vi "Stage position constant read.vi"(11 "Queue in":refnum<queue>) -> ()   [LabVIEW 2020]
panel:
  out "Stage position":dbl format="%.1f"
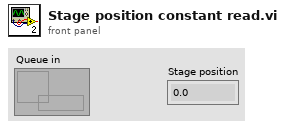
[diagram p1: front panel]
types:
  T1 = enum32{"invalid app kind", "Development System", "Run Time System", "Student Edition", "Embedded LabVIEW", "Evaluation", "Custom"}
  T2 = enum32{"Invalid", "Standard", "Closed", "Hidden", "Minimized", "Maximized"}
  T3 = cluster{"Core":cluster{"Current VI Reference":refnum<vi>, "Close Panel on Exit?":bool}, "Stage name":string, "Stage variable name":string, "Stage TCP":refnum<k5>, "Stage status":cluster{"stage position":dbl, "display error":bool}, "connected":bool}
  T4 = cluster{"stage position":dbl, "display error":bool}
  T5 = cluster{"Current VI Reference":refnum<vi>, "Close Panel on Exit?":bool}
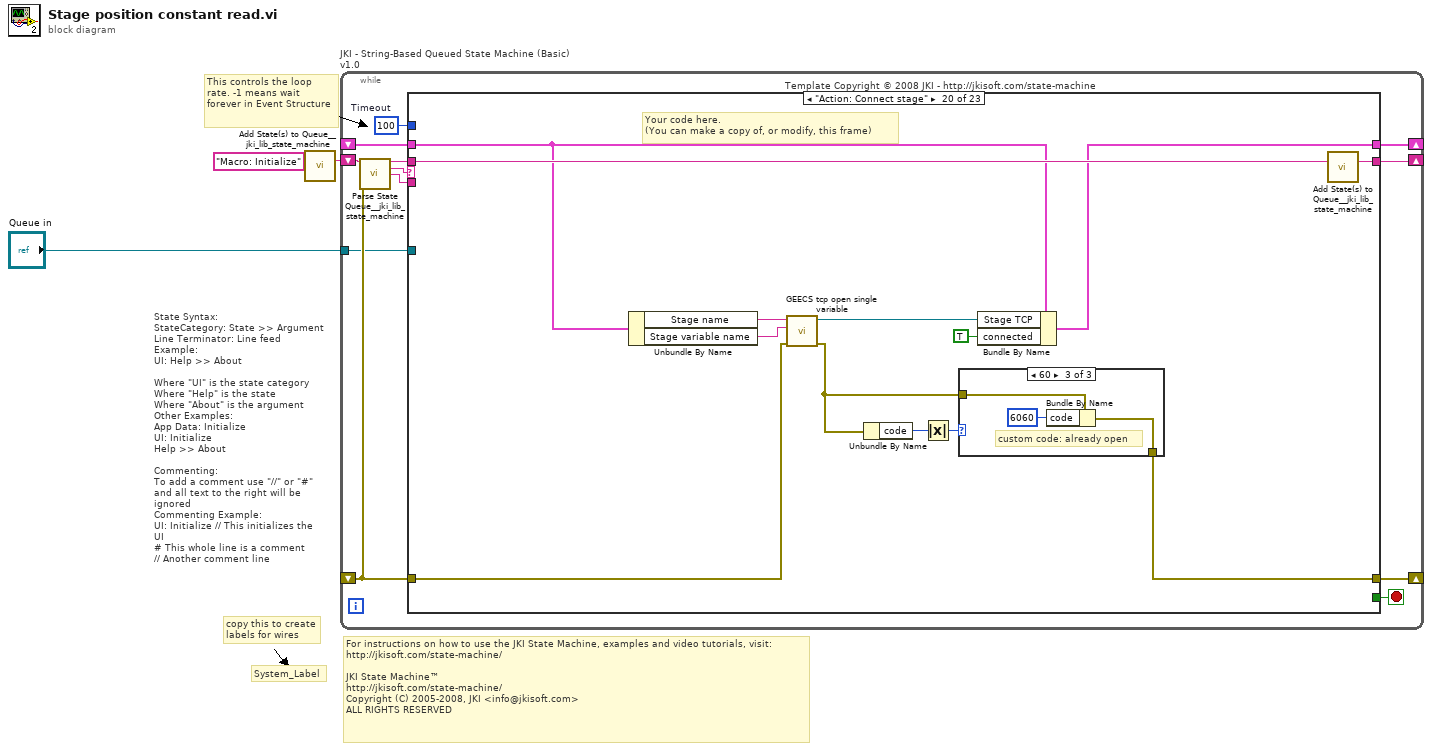
[diagram p0: block diagram]
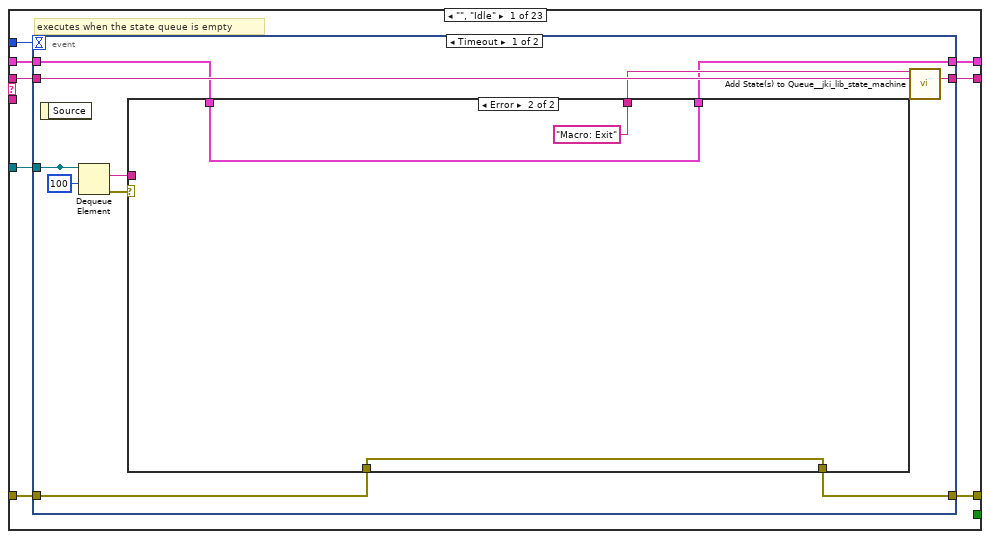
[diagram p2: hidden frame]
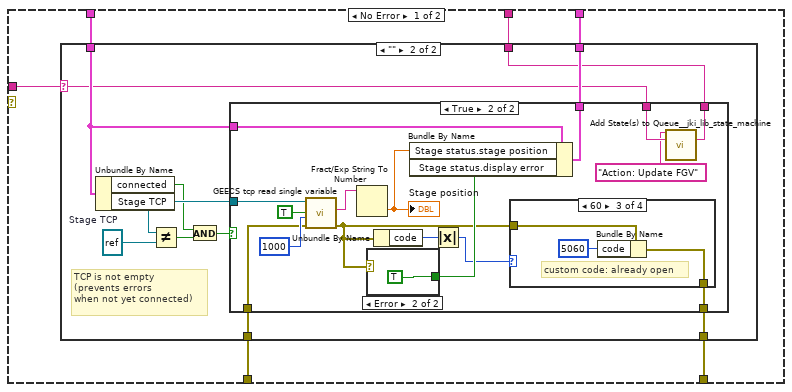
[diagram p3: hidden frame]
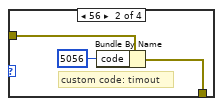
[diagram p7: hidden frame]
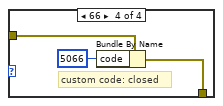
[diagram p8: hidden frame]
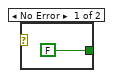
[diagram p9: hidden frame]
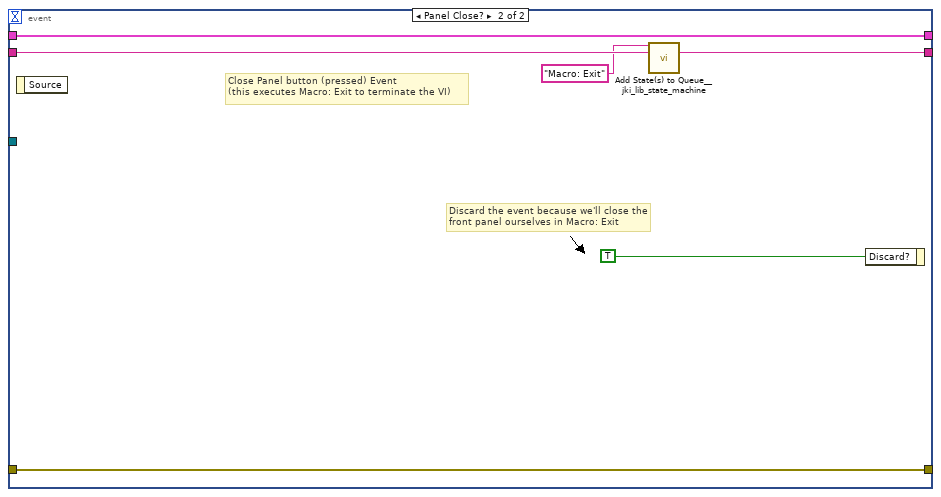
[diagram p10: hidden frame]
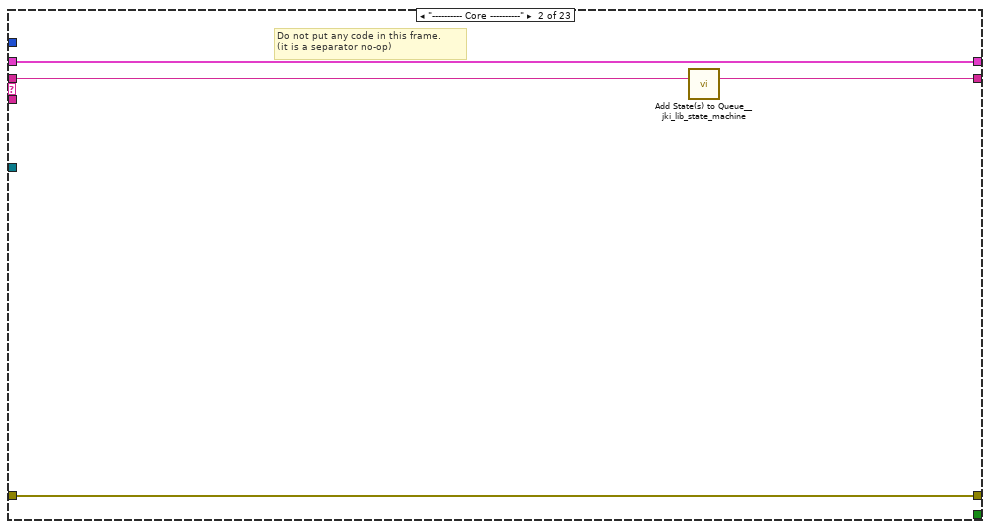
[diagram p11: hidden frame]
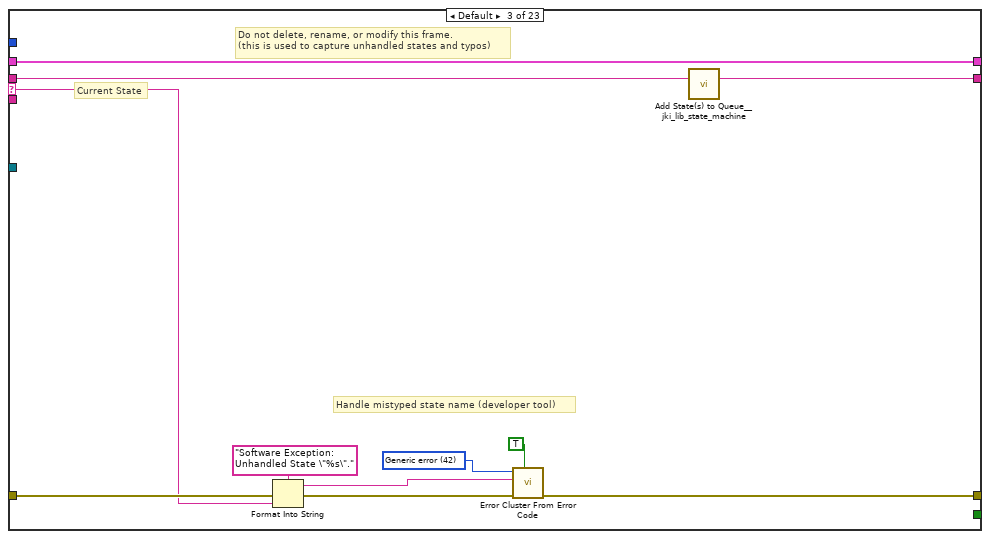
[diagram p12: hidden frame]
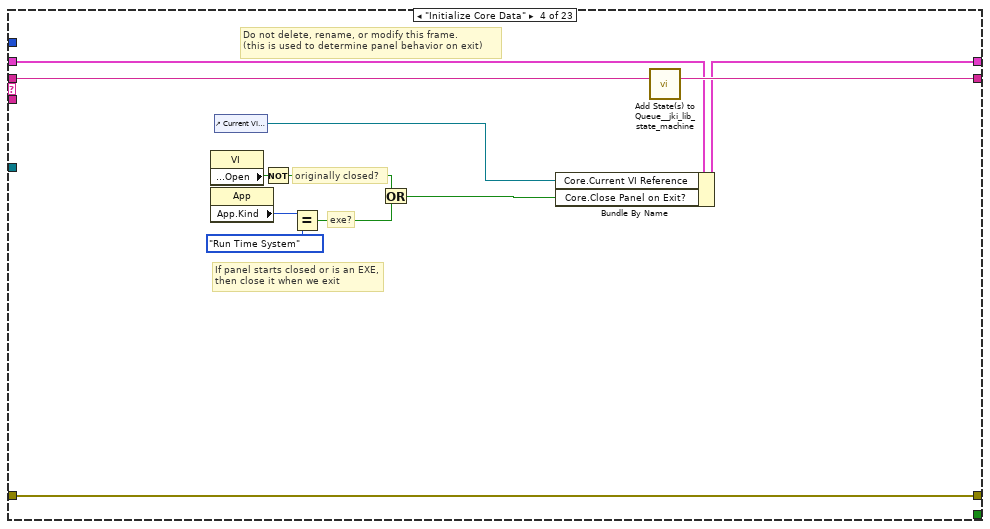
[diagram p13: hidden frame]
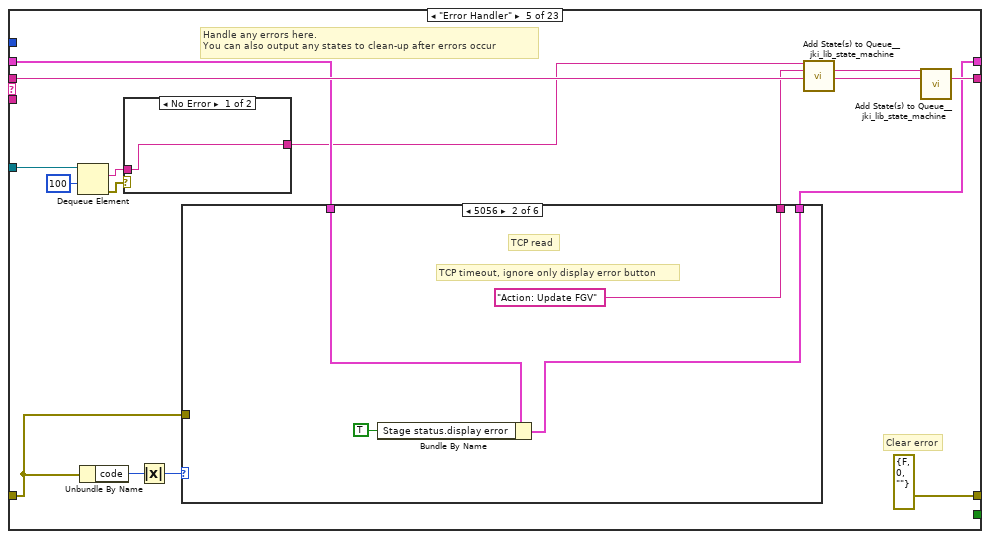
[diagram p14: hidden frame]
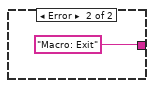
[diagram p15: hidden frame]
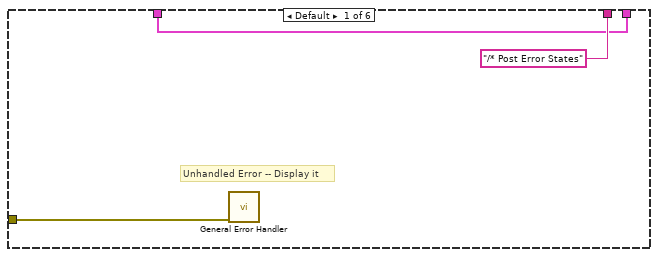
[diagram p16: hidden frame]
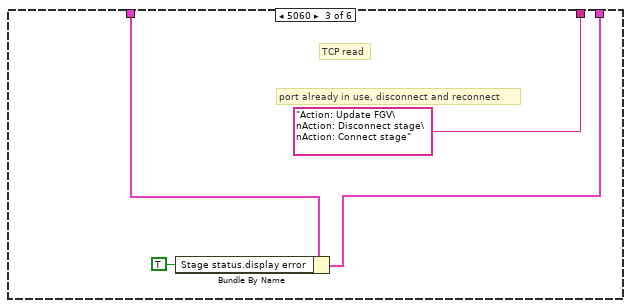
[diagram p17: hidden frame]
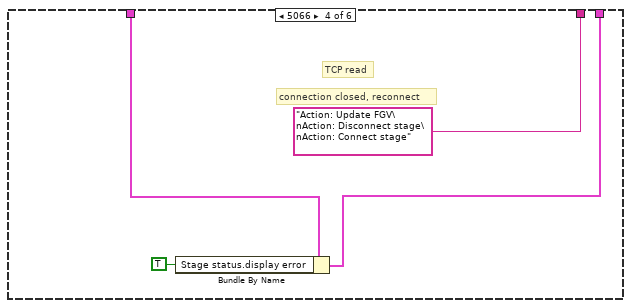
[diagram p18: hidden frame]
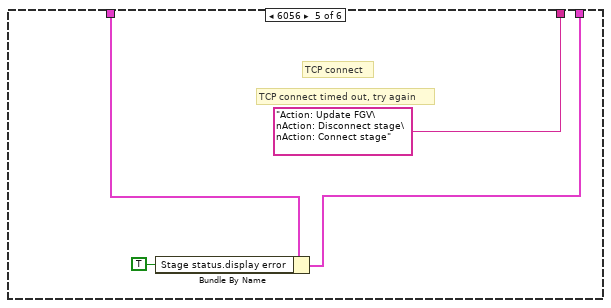
[diagram p19: hidden frame]
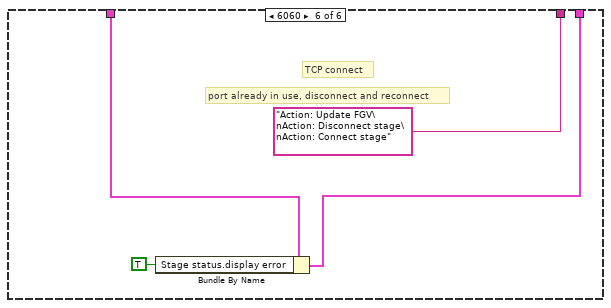
[diagram p20: hidden frame]
diagram:
  # "For instructions on how to use the JKI State Machine, examples and video tutorials, visit:\nhttp://jkisoft.com/state-machine/\n\nJKI State Machine™\nhttp://jkisoft.com/state-machine/\nCopyright (C) 2005-2008, JKI <info@jkisoft.com>\nALL RIGHTS RESERVED"
  # "State Syntax:\nStateCategory: State >> Argument\nLine Terminator: Line feed\nExample:\nUI: Help >> About\n\nWhere \"UI\" is the state category\nWhere \"Help\" is the state\nWhere \"About\" is the argument\nOther Examples:\nApp Data: Initialize\nUI: Initialize\nHelp >> About\n\nCommenting:\nTo add a comment use \"//\" or \"#\" and all text to the right will be ignored\nCommenting Example:\nUI: Initialize // This initializes the UI\n# This whole line is a comment\n// Another comment line"
  # "copy this to create labels for wires"
  # "This controls the loop rate. -1 means wait forever in Event Structure"
  # "System_Label"
  n1 = call <vilib>:"Add State(s) to Queue__jki_lib_state_machine.vi"("State(s) in (\"\")"="Macro: Initialize") -> ("States Out"=w3:string)  [unwired: 14 in]
  n2 = while "JKI - String-Based Queued State Machine (Basic) v1.0" {
    shift-right: [w8] -> _
    shift-left: _ -> [w7]
    shift-right: [w11] -> _
    shift-left: _ -> [w5]
    shift-right: [w10] -> _
    shift-left: w3 -> [w12]
    tunnel: "Queue in" -> [w4]
    stop <- w9 stop-if-true
    w6 = 100  # Timeout
    # "Template Copyright © 2008 JKI - http://jkisoft.com/state-machine"
    n3 = call <vilib>:"Parse State Queue__jki_lib_state_machine.vi"("State Queue"=w12, "Error In (no error)"=w5) -> ("Remaining States"=w14:string, "Current State"=w15:string, "Arguments"=w13:string)  [unwired: 11 in]
    n4 = case shown="\"Action: Connect stage\"" w15 {
      selector: w15 -> [_ _ w99 _ _ _ _ _ _ _ _ _ _ _ _ _ _ _ _ _ _ _ _]
      tunnel: w14 -> [w23 w98 w103 w121 w136 w166 w170 w180 w186 w190 w194 w200 w211 w237 w242 w253 w257 w265 w269 w282 w297 w303 w307]
      tunnel: w13 -> [_ _ _ _ _ _ _ _ _ _ _ w195 w205 _ _ _ _ w262 _ _ _ _ _]
      tunnel: w7 -> [w21 w95 w101 w112 w131 w164 w167 _ w181 w187 w192 w198 w207 w234 w239 w250 w254 w261 w266 w278 w292 w298 w304]
      tunnel: [w20 w96 w105 w118 errorcluster {"status"=FALSE, "code"=0, "source"=""} ("error out") w163 w168 w177 w182 w188 w191 w196 w208 w235 w240 w251 w255 w263 w267 w273 w295 w301 w305] -> w11
      tunnel: w5 -> [w19 w96 w104 w118 w132 w163 w168 w177 w183 w188 w191 w197 w209 w235 w240 w251 w255 w263 w267 w275 w295 w301 w305]
      tunnel: [w22 w97 w102 w120 w135 w165 w169 w179 w185 w189 w193 w199 w210 w236 w241 w252 w256 w264 w268 w281 w296 w302 w306] -> w10
      tunnel: [_ _ _ _ _ TRUE _ _ _ _ _ _ _ _ _ _ _ _ _ _ _ _ _] -> w9
      tunnel: [w18 w95 w101 w119 w130 w164 w167 w178 w181 w187 w192 w198 w207 w234 w239 w250 w254 w260 w266 w277 w291 w298 w304] -> w8
      tunnel: w6 -> [w17 _ _ _ _ _ _ _ _ _ _ _ _ _ _ _ _ _ _ _ _ _ _]
      tunnel: w4 -> [w16 _ _ _ w127 _ _ _ _ _ _ _ _ _ _ _ _ _ _ _ _ _ _]
      frame "", "Idle" {
        # "executes when the state queue is empty"
        n5 = event shown="[0] Timeout" {
          selector: _ -> [_ _]
          dyn-events: _ -> [_ _]
          timeout: w17 -> [_ _]
          tunnel: w23 -> [w34 w94]
          tunnel: [w33 w93] -> w22
          tunnel: w21 -> [w25 w91]
          tunnel: [w26 w92] -> w20
          tunnel: w19 -> [w27 w92]
          tunnel: [w24 w91] -> w18
          tunnel: [w32 _] -> _
          tunnel: w16 -> [w32 _]
          event Timeout {
            n6 = event-data() -> ()  [unwired: 1 in, 1 out]
            n7 = Dequeue Element(queue=w32, timeout in ms (-1)=100) -> (element=w28:string, error out=w30:errorcluster)  [unwired: 1 in, 2 out]
            n8 = case shown="Error" w30 {
              tunnel: [w35 "Macro: Exit"] -> w29
              tunnel: w28 -> [w36 _]
              tunnel: w25 -> [w40 w86]
              tunnel: w27 -> [w39 w87]
              tunnel: [w38 w87] -> w26
              tunnel: [w37 w86] -> w24
              frame No Error {
                n9 = case shown="\"\"" w36 {
                  selector: w36 -> [w43 w48]
                  tunnel: w40 -> [w41 w49]
                  tunnel: w39 -> [w42 w54]
                  tunnel: [w42 w53] -> w38
                  tunnel: [w41 w50] -> w37
                  tunnel: [w43 w47] -> w35
                  frame Default {
                  }
                  frame "" {
                    w52 = refnum<k5> refnum  # Stage TCP
                    # "TCP is not empty\n(prevents errors \nwhen not yet connected)"
                    n10 = Unbundle By Name(w49) -> ("connected"=w45:bool, "Stage TCP"=w51:refnum<k5>)
                    n11 = Not Equal?(x=w51, y=w52) -> (x != y?=w46:bool)
                    n12 = And(x=w45, y=w46) -> (x .and. y?=w44:bool)
                    n13 = case shown="True" w44 {
                      tunnel: w51 -> [_ w71]
                      tunnel: w54 -> [w57 w70]
                      tunnel: [w57 w59] -> w53
                      tunnel: [w56 w67] -> w50
                      tunnel: w49 -> [w56 w66]
                      tunnel: w48 -> [w55 w65]
                      tunnel: [w55 w64] -> w47
                      frame False {
                      }
                      frame True {
                        n14 = call "GEECS tcp read single variable.vi"("error in (no error)"=w70, "timeout ms (2000)"=1000, "clear buffer after read"=TRUE, "TCP Network Connection in"=w71) -> ("error out"=w58:errorcluster, "variable value"=w69:string)  [unwired: 4 in, 2 out]
                        n15 = Fract/Exp String To Number(string=w69) -> (number=w68:dbl)  [unwired: 3 in, 1 out]
                        "Stage position" <- w68
                        n16 = case shown="Error" w58 {
                          tunnel: [FALSE TRUE] -> w62
                          frame No Error {
                          }
                          frame Error {
                          }
                        }
                        n17 = Unbundle By Name(w58) -> ("code"=w61:i32)
                        n18 = Bundle By Name(cluster=w66, "Stage status.stage position"=w68, "Stage status.display error"=w62) -> (w67:T3)
                        n19 = Absolute Value(x=w61) -> (abs(x)=w60:i32)
                        n20 = case shown="60" w60 {
                          tunnel: [w74 w76 w79 w82] -> w59
                          tunnel: w58 -> [w74 w77 w80 w83]
                          frame Default {
                          }
                          frame 56 {
                            # "custom code: timout"
                            n21 = Bundle By Name(cluster=w77, "code"=5056) -> (w76:errorcluster)
                          }
                          frame 60 {
                            # "custom code: already open"
                            n22 = Bundle By Name(cluster=w80, "code"=5060) -> (w79:errorcluster)
                          }
                          frame 66 {
                            # "custom code: closed"
                            n23 = Bundle By Name(cluster=w83, "code"=5066) -> (w82:errorcluster)
                          }
                        }
                        n24 = call <vilib>:"Add State(s) to Queue__jki_lib_state_machine.vi"("State(s) in Front (\"\")"="Action: Update FGV" ("State(s) at Back (\"\")"), "State(s) in (\"\")"=w65) -> ("States Out"=w64:string)  [unwired: 13 in]
                      }
                    }
                  }
                }
              }
              frame Error {
              }
            }
            n25 = call <vilib>:"Add State(s) to Queue__jki_lib_state_machine.vi"("State(s) in Front (\"\")"=w29, "State(s) in (\"\")"=w34) -> ("States Out"=w33:string)  [unwired: 13 in]
          }
          event Panel Close? {
            # "Discard the event because we'll close the front panel ourselves in Macro: Exit"
            # "Close Panel button (pressed) Event\n(this executes Macro: Exit to terminate the VI)"
            n26 = event-data() -> ()  [unwired: 1 in, 1 out]
            n27 = call <vilib>:"Add State(s) to Queue__jki_lib_state_machine.vi"("State(s) in Front (\"\")"="Macro: Exit", "State(s) in (\"\")"=w94) -> ("States Out"=w93:string)  [unwired: 13 in]
            n28 = event-data("Discard?"=TRUE) -> ()  [unwired: 1 in, 1 out]
          }
        }
      }
      frame "---------- Core ----------" {
        # "Do not put any code in this frame.\n(it is a separator no-op)"
        n29 = call <vilib>:"Add State(s) to Queue__jki_lib_state_machine.vi"("State(s) in (\"\")"=w98) -> ("States Out"=w97:string)  [unwired: 14 in]
      }
      frame Default {
        w108 = 42 items=["No error", "Argument error", "Memory is full", "Out of zone", "End of file", "File already open", "Generic file I/O error", "File not found", "File permission error", "Disk is full", "Duplicate path", "Too many files open", "System feature not enabled", "Resource file not found", "Cannot add resource", "Resource not found", "Image not found", "Image memory error", "Pen does not exist", "Config type invalid", "Config token not found", "Config parse error", "Config memory error", "Bad external code format", "Bad external code offset", "External code not present", "Null window", "Destroy window error", "Null menu", "Print aborted", "Bad print record", "Print driver error", "Windows error during printing", "Memory error during printing", "Print dialog error", "Generic print error", "Invalid device refnum", "Device not found", "Device parameter error", "Device unit error", "Cannot open device", "Device call aborted", "Generic error", "Cancelled by user", "Object ID too low", "Object ID too high", "Object not in heap", "Unknown heap", "Unknown object (invalid DefProc)", "Unknown object (DefProc not in table)", "Message out of range", "Invalid (null) method", "Unknown message", "Manager call not supported", "Bad address", "Network operation in progress", "Network operation timed out", "Connection is busy", "Network attribute not supported", "Network error", "Address in use", "System out of memory", "Connection aborted", "Connection refused", "Not connected", "Already connected", "Connection closed", "Initialization error (interapplication manager)", "Bad occurrence", "Wait on unbound occurrence handler", "Occurrence queue overflow", "Datalog type conflict", "Unused", "Unrecognized type (interapplication manager)", "Memory corrupt", "Failed to make temporary DLL", "Old CIN version", "Drag socket not found", "Failed to load drop-object", "Failed to register OLE object", "Failed to release OLE object", "Format specifier type mismatch", "Unknown format specifier", "Too few format specifiers", "Too many format specifiers", "Scan failed", "Newer CIN version", "Error converting to variant", "Runtime menu error", "Password tampered", "Variant attribute not found", "Incompatible variant data type", "Event data is not available", "Event Store is not present", "Occurrence is not found", "Event Queue is not created", "Event info is not available", "Refnum passed is NULL", "Error retrieving Class GUID", "Error retrieving CoClass GUID", "Error retrieving TypeLib GUID.", "Bad built application magic bytes.", "Specific driver is different from the specific driver associated with the Logical Name.", "There is no session opened to the class driver.", "Max Error", "MAX - Error with config objects", "MAX - Error loading configuration", "MAX - Group not supported"]
        # "Current State"
        # "Do not delete, rename, or modify this frame.\n(this is used to capture unhandled states and typos)"
        # "Handle mistyped state name (developer tool)"
        n30 = Format Into String(format string="Software Exception: Unhandled State \"%s\"." ("message"), error in=w104, w99) -> (resulting string=w107:string, error out=w106:errorcluster)  [unwired: 1 in]
        n31 = call <vilib>:"Error Cluster From Error Code.vi"("show call chain? (False)"=TRUE, "error in (no error)"=w106, "error message (\"\")"=w107, "error code (0)"=w108) -> ("error out"=w105:errorcluster)  [unwired: 5 in]
        n32 = call <vilib>:"Add State(s) to Queue__jki_lib_state_machine.vi"("State(s) in (\"\")"=w103) -> ("States Out"=w102:string)  [unwired: 14 in]
      }
      frame "Initialize Core Data" {
        # "Do not delete, rename, or modify this frame.\n(this is used to determine panel behavior on exit)"
        # "originally closed?"
        # "exe?"
        # "If panel starts closed or is an EXE, then close it when we exit"
        n33 = property class="VI"() -> ("Front Panel.Open"=w117:bool)  [unwired: 2 in, 2 out]
        n34 = property class="App"() -> ("App.Kind"=w116:T1)  [unwired: 2 in, 2 out]
        n35 = control-ref of="Current VI Reference"() -> (w110:refnum<vi>)
        n36 = Not(x=w117) -> (.not. x?=w114:bool)
        n37 = Equal?(x=w116, y=T1."Run Time System" ("Application:Kind")) -> (x = y?=w113:bool)
        n38 = Or(x=w114, y=w113) -> (x .or. y?=w111:bool)
        n39 = Bundle By Name(cluster=w112, "Core.Current VI Reference"=w110, "Core.Close Panel on Exit?"=w111) -> (w119:T3)
        n40 = call <vilib>:"Add State(s) to Queue__jki_lib_state_machine.vi"("State(s) in (\"\")"=w121) -> ("States Out"=w120:string)  [unwired: 14 in]
      }
      frame "Error Handler" {
        # "Handle any errors here.\nYou can also output any states to clean-up after errors occur"
        # "Clear error"
        n41 = Dequeue Element(queue=w127, timeout in ms (-1)=100) -> (element=w125:string, error out=w126:errorcluster)  [unwired: 1 in, 2 out]
        n42 = Unbundle By Name(w132) -> ("code"=w133:i32)
        n43 = case shown="No Error" w126 {
          tunnel: w125 -> [w137 _]
          tunnel: [w137 "Macro: Exit"] -> w122
          frame No Error {
          }
          frame Error {
          }
        }
        n44 = Absolute Value(x=w133) -> (abs(x)=w129:i32)
        n45 = case shown="5056" w129 {
          tunnel: w132 -> [w141 _ _ _ _ _]
          tunnel: ["/* Post Error States" "Action: Update FGV" "Action: Update FGV\nAction: Disconnect stage\nAction: Connect stage" "Action: Update FGV\nAction: Disconnect stage\nAction: Connect stage" "Action: Update FGV\nAction: Disconnect stage\nAction: Connect stage" "Action: Update FGV\nAction: Disconnect stage\nAction: Connect stage"] -> w123
          tunnel: w131 -> [w139 w143 w148 w152 w156 w160]
          tunnel: [w139 w142 w147 w151 w155 w159] -> w130
          frame Default {
            # "Unhandled Error -- Display it"
            n46 = call <vilib>:"General Error Handler.vi"("error in (no error)"=w141) -> ()  [unwired: 10 in, 5 out]
          }
          frame 5056 {
            # "TCP read"
            # "TCP timeout, ignore only display error button"
            n47 = Bundle By Name(cluster=w143, "Stage status.display error"=TRUE) -> (w142:T3)
          }
          frame 5060 {
            # "TCP read"
            # "port already in use, disconnect and reconnect"
            n48 = Bundle By Name(cluster=w148, "Stage status.display error"=TRUE) -> (w147:T3)
          }
          frame 5066 {
            # "TCP read"
            # "connection closed, reconnect"
            n49 = Bundle By Name(cluster=w152, "Stage status.display error"=TRUE) -> (w151:T3)
          }
          frame 6056 {
            # "TCP connect"
            # "TCP connect timed out, try again"
            n50 = Bundle By Name(cluster=w156, "Stage status.display error"=TRUE) -> (w155:T3)
          }
          frame 6060 {
            # "port already in use, disconnect and reconnect"
            # "TCP connect"
            n51 = Bundle By Name(cluster=w160, "Stage status.display error"=TRUE) -> (w159:T3)
          }
        }
        n52 = call <vilib>:"Add State(s) to Queue__jki_lib_state_machine.vi"("State(s) in Front (\"\")"=w122, "State(s) in (\"\")"=w123) -> ("States Out"=w124:string)  [unwired: 13 in]
        n53 = call <vilib>:"Add State(s) to Queue__jki_lib_state_machine.vi"("State(s) in Front (\"\")"=w124, "State(s) in (\"\")"=w136) -> ("States Out"=w135:string)  [unwired: 13 in]
      }
      frame "Exit" {
        # "Do not put any code in this frame.\n(No errors that occur here will be handled.)"
        n54 = call <vilib>:"Add State(s) to Queue__jki_lib_state_machine.vi"("State(s) in (\"\")"=w166) -> ("States Out"=w165:string)  [unwired: 14 in]
      }
      frame "---------- Data ----------" {
        # "Do not put any code in this frame.\n(It is a separator no-op. You can make a copy of this frame to create a new Data frame)"
        n55 = call <vilib>:"Add State(s) to Queue__jki_lib_state_machine.vi"("State(s) in (\"\")"=w170) -> ("States Out"=w169:string)  [unwired: 14 in]
      }
      frame "Data: Initialize" {
        w171 = FALSE  # connected
        w172 = T4 {"stage position"=0.0, "display error"=FALSE}  # Stage status
        w173 = refnum<k5> refnum  # Stage TCP
        w174 = ""  # Stage variable name
        w175 = ""  # Stage name
        w176 = T5 {"Current VI Reference"=refnum, "Close Panel on Exit?"=FALSE}  # Core
        # "do not delete - used by framework"
        # "Initialize the shift-register data, here.\n(data names are defined by what you wire into the bundle function)"
        n56 = Bundle("Core"=w176, "Stage name"=w175, "Stage variable name"=w174, "Stage TCP"=w173, "Stage status"=w172, "connected"=w171) -> (w178:T3)  [unwired: 1 in]
        n57 = call <vilib>:"Add State(s) to Queue__jki_lib_state_machine.vi"("State(s) in (\"\")"=w180) -> ("States Out"=w179:string)  [unwired: 14 in]
      }
      frame "Data: Cleanup" {
        # "Cleanup any data and references, here.\n(this is called automatically, by the Macro: Exit)"
        n58 = Unbundle By Name(w181) -> ("Core.Current VI Reference"=w184:refnum<vi>)
        n59 = Close Reference(reference=w184, error in (no error)=w183) -> (error out=w182:errorcluster)
        n60 = call <vilib>:"Add State(s) to Queue__jki_lib_state_machine.vi"("State(s) in (\"\")"=w186) -> ("States Out"=w185:string)  [unwired: 14 in]
      }
      frame "---------- UI ----------" {
        # "Do not put any code in this frame.\n(It is a separator no-op. You can make a copy of this frame to create a new UI frame)"
        n61 = call <vilib>:"Add State(s) to Queue__jki_lib_state_machine.vi"("State(s) in (\"\")"=w190) -> ("States Out"=w189:string)  [unwired: 14 in]
      }
      frame "UI: Initialize" {
        # "Initialize the User Interface, here.\n(this is called automatically, by the Macro: Init)"
        n62 = call <vilib>:"Add State(s) to Queue__jki_lib_state_machine.vi"("State(s) in (\"\")"=w194) -> ("States Out"=w193:string)  [unwired: 14 in]
      }
      frame "UI: Cursor Set" {
        # "Argument"
        # "Set and Unset Cursor Busy.\n(Usage: \"UI: Cursor Set >> Busy|Idle\")"
        n63 = case shown="\"Idle\", Default" w195 {
          tunnel: w197 -> [w202 w204]
          tunnel: [w201 w203] -> w196
          frame "Idle", Default {
            n64 = call <vilib>:"Unset Busy.vi"("error in (no error)"=w202) -> ("error out"=w201:errorcluster)  [unwired: 10 in]
          }
          frame "Busy" {
            n65 = call <vilib>:"Set Busy.vi"("error in (no error)"=w204) -> ("error out"=w203:errorcluster)  [unwired: 9 in, 1 out]
          }
        }
        n66 = call <vilib>:"Add State(s) to Queue__jki_lib_state_machine.vi"("State(s) in (\"\")"=w200) -> ("States Out"=w199:string)  [unwired: 14 in]
      }
      frame "UI: Front Panel State" {
        # "Argument"
        # "Set Front Panel Open or Closed\n(Usage: \"UI: Front Panel State >> Open|Close\")"
        n67 = Unbundle By Name(w207) -> ("Core.Current VI Reference"=w206:refnum<vi>)
        n68 = case shown="\"Open\", Default" w205 {
          tunnel: w209 -> [w215 w228]
          tunnel: [w217 w229] -> w208
          tunnel: w206 -> [w216 w226]
          frame "Open", Default {
            n69 = property class="VI"(reference=w216, error in=w215) -> (reference out=w213:refnum<vi>, error out=w214:errorcluster, "Front Panel.Open"=w212:bool)
            n70 = case shown="False" w212 {
              tunnel: [w220 w223] -> w217
              tunnel: w214 -> [w219 w223]
              tunnel: w213 -> [w218 _]
              frame False {
                n71 = invoke class="VI" method="FP.Open"(reference=w218, error in=w219, "Activate"=TRUE, "State"=T2."Standard") -> (error out=w220:errorcluster)  [unwired: 1 in, 4 out]
              }
              frame True {
              }
            }
          }
          frame "Close" {
            n72 = property class="VI"(reference=w226, error in=w228) -> (reference out=w225:refnum<vi>, error out=w227:errorcluster, "Front Panel.Open"=w224:bool)
            n73 = case shown="True" w224 {
              tunnel: [w230 w233] -> w229
              tunnel: w227 -> [w230 w232]
              tunnel: w225 -> [_ w231]
              frame False {
              }
              frame True {
                n74 = invoke class="VI" method="FP.Close"(reference=w231, error in=w232) -> (error out=w233:errorcluster)  [unwired: 1 in, 2 out]
              }
            }
          }
        }
        n75 = call <vilib>:"Add State(s) to Queue__jki_lib_state_machine.vi"("State(s) in (\"\")"=w211) -> ("States Out"=w210:string)  [unwired: 14 in]
      }
      frame "---------- Macro ----------" {
        # "Do not put any code in this frame.\n(It is a separator no-op. You can make a copy of this frame to create a new Macro frame)"
        n76 = call <vilib>:"Add State(s) to Queue__jki_lib_state_machine.vi"("State(s) in (\"\")"=w237) -> ("States Out"=w236:string)  [unwired: 14 in]
      }
      frame "Macro: Initialize" {
        (unwired) "Data: Initialize\nInitialize Core Data\nUI: Initialize\nUI: Front Panel State >> Open"  # Data: Initialize Initialize Core Data UI: Initialize UI: Front Panel State >> Open
        # "Initialization Macro\n(This is called once, when the VI starts)"
        n77 = call <vilib>:"Add State(s) to Queue__jki_lib_state_machine.vi"("State(s) in Front (\"\")"="Data: Initialize\nInitialize Core Data\nUI: Initialize", "State(s) in (\"\")"=w242) -> ("States Out"=w241:string)  [unwired: 13 in]
      }
      frame "Macro: Exit" {
        # "Exit Macro\n(This is called once, when the VI exits)"
        n78 = Unbundle By Name(w250) -> ("Core.Close Panel on Exit?"=w249:bool)
        n79 = Select(t="UI: Front Panel State >> Close", s=w249, f="") -> (s? t:f=w246:string)
        n80 = call <vilib>:"Add State(s) to Queue__jki_lib_state_machine.vi"("State(s) in Front (\"\")"="Action: Disconnect stage", "State(s) in (\"\")"=w246, "State(s) at Back (\"\")"="Data: Cleanup\nExit") -> ("States Out"=w244:string)  [unwired: 12 in]
        n81 = call <vilib>:"Add State(s) to Queue__jki_lib_state_machine.vi"("State(s) in Front (\"\")"=w244, "State(s) in (\"\")"=w253) -> ("States Out"=w252:string)  [unwired: 13 in]
      }
      frame "---------- Main actions ----------" {
        # "Template Separator\n(You can make a copy of, or modify, this frame)"
        n82 = call <vilib>:"Add State(s) to Queue__jki_lib_state_machine.vi"("State(s) in (\"\")"=w257) -> ("States Out"=w256:string)  [unwired: 14 in]
      }
      frame "Main action: Set stage name" {
        # "Your code here.\n(You can make a copy of, or modify, this frame)"
        n83 = call "get arguments of jki state.vi"("jki arguments"=w262) -> ("Arg 1"=w259:string, "Arg 2"=w258:string)  [unwired: 1 in, 1 out]
        n84 = Bundle By Name(cluster=w261, "Stage name"=w259, "Stage variable name"=w258) -> (w260:T3)
        n85 = call <vilib>:"Add State(s) to Queue__jki_lib_state_machine.vi"("State(s) in (\"\")"=w265) -> ("States Out"=w264:string)  [unwired: 14 in]
      }
      frame "---------- Actions ----------" {
        # "Template Separator\n(You can make a copy of, or modify, this frame)"
        n86 = call <vilib>:"Add State(s) to Queue__jki_lib_state_machine.vi"("State(s) in (\"\")"=w269) -> ("States Out"=w268:string)  [unwired: 14 in]
      }
      frame "Action: Connect stage" {
        # "Your code here.\n(You can make a copy of, or modify, this frame)"
        n87 = Unbundle By Name(w278) -> ("Stage name"=w279:string, "Stage variable name"=w280:string)
        n88 = call "GEECS tcp open single variable.vi"("error in (no error)"=w275, "Variable name"=w280, "Device name"=w279) -> ("error out"=w270:errorcluster, "TCP Network Connection out"=w276:refnum<k5>)  [unwired: 6 in, 1 out]
        n89 = Unbundle By Name(w270) -> ("code"=w271:i32)
        n90 = Absolute Value(x=w271) -> (abs(x)=w272:i32)
        n91 = case shown="60" w272 {
          tunnel: [w283 w285 w288] -> w273
          tunnel: w270 -> [w283 w286 w289]
          frame Default {
          }
          frame 56 {
            # "custom code: timout"
            n92 = Bundle By Name(cluster=w286, "code"=6056) -> (w285:errorcluster)
          }
          frame 60 {
            # "custom code: already open"
            n93 = Bundle By Name(cluster=w289, "code"=6060) -> (w288:errorcluster)
          }
        }
        n94 = Bundle By Name(cluster=w278, "Stage TCP"=w276, "connected"=TRUE) -> (w277:T3)
        n95 = call <vilib>:"Add State(s) to Queue__jki_lib_state_machine.vi"("State(s) in (\"\")"=w282) -> ("States Out"=w281:string)  [unwired: 14 in]
      }
      frame "Action: Disconnect stage" {
        # "variable to prevent\nthe idle case from trying to keep reading the\nstage position"
        # "Your code here.\n(You can make a copy of, or modify, this frame)"
        n96 = Unbundle By Name(w292) -> ("Stage TCP"=w294:refnum<k5>)
        n97 = TCP Close Connection(connection ID=w294) -> (error out=w293:errorcluster)  [unwired: 2 in, 1 out]
        n98 = call <vilib>:"Clear Errors.vi"("error in (no error)"=w293) -> ()  [unwired: 5 in, 2 out]
        n99 = Bundle By Name(cluster=w292, "connected"=FALSE) -> (w291:T3)
        n100 = call <vilib>:"Add State(s) to Queue__jki_lib_state_machine.vi"("State(s) in (\"\")"=w297) -> ("States Out"=w296:string)  [unwired: 14 in]
      }
      frame "Action: Update FGV" {
        # "Your code here.\n(You can make a copy of, or modify, this frame)"
        n101 = Unbundle By Name(w298) -> ("Stage status"=w299:T4)
        n102 = call "Stage position FGV.vi"("Stage status (in)"=w299, "Action"=enum16{"read", "write", "clear"}."write") -> ()  [unwired: 9 in, 1 out]
        n103 = call <vilib>:"Add State(s) to Queue__jki_lib_state_machine.vi"("State(s) in (\"\")"=w303) -> ("States Out"=w302:string)  [unwired: 14 in]
      }
      frame "Duplicate me" {
        # "Your code here.\n(You can make a copy of, or modify, this frame)"
        n104 = call <vilib>:"Add State(s) to Queue__jki_lib_state_machine.vi"("State(s) in (\"\")"=w307) -> ("States Out"=w306:string)  [unwired: 14 in]
      }
    }
  }
